vi "Addition.vi"() -> ()   [LabVIEW 2020]
panel:
  in  "Boolean":bool
  out "x+y":dbl
  in  "y":dbl
  in  "x":dbl
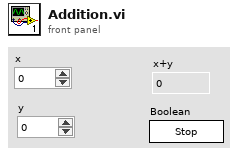
[diagram p1: front panel]
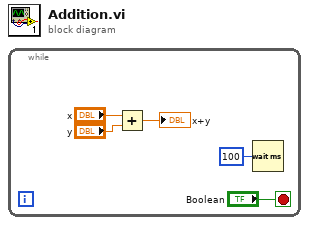
[diagram p0: block diagram]
diagram:
  n1 = while {
    stop <- "Boolean" stop-if-true
    n2 = Add(x="x", y="y") -> (x+y=→"x+y":dbl)
    n3 = Wait (ms)(milliseconds to wait=u32 100) -> ()  [unwired: 1 out]
  }
